vi "axex_write_cells_vector.vi"(7 "vertical vector (False)":bool, 8 "error in":errorcluster, 9 "strings vector":string[](array[string]), 10 "top-left cell":T1, 11 "AX Excel instance in":T2) -> (0 "error out":errorcluster, 3 "AX Excel instance out":T2)   [LabVIEW 2020, in "AX Excel.lvlib"]
doc: "Call this to write vector of string to cells. The coordinates of top-left cell may be given as [column,row] index or cell name such as A1, AB66, ... with priority of cell name."
uses:
  AX Excel.lvlib
  axex_instance.ctl
  axex_cell_xy.ctl
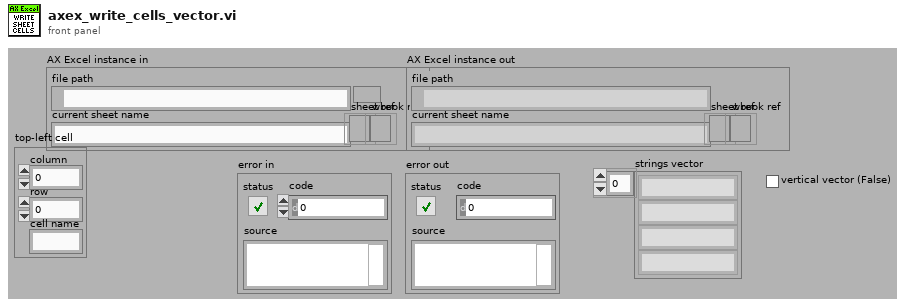
[diagram p1: front panel]
types:
  T1 = typedef "AX Excel.lvlib/axex_cell_xy.ctl" = cluster{"column":i32, "row":i32, "cell name":string}
  T2 = typedef "AX Excel.lvlib/axex_instance.ctl" = cluster{"file path":path, "current sheet name":string, "sheet ref":refnum<k7>, "wbook ref":refnum<k7>}
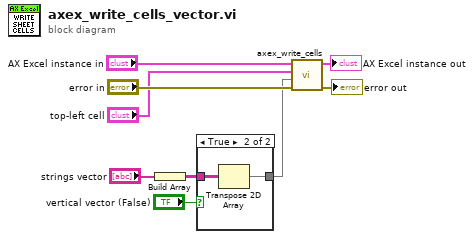
[diagram p0: block diagram]
diagram:
  n1 = Build Array("strings vector") -> (w2:string[][])
  n2 = case shown="True" "vertical vector (False)" {
    tunnel: w2 -> [w10 w12]
    tunnel: [w10 w11] -> w1
    frame False {
    }
    frame True {
      n3 = Transpose 2D Array(2D array=w12) -> (transposed array=w11:string[][])
    }
  }
  n4 = call "axex_write_cells.vi"("error in"="error in", "cell array"=w1, "top left cell"="top-left cell", "AX Excel instance in"="AX Excel instance in") -> ("error out"=→"error out":errorcluster, "AX Excel instance out"=→"AX Excel instance out":T2)  [unwired: 6 in]
